vi "Vision on GIC Lab.vi"(11 "GIC Input":T2={"Real/Sim"=FALSE, "WP Lats and Longs"={"WP Lats"=[], "WP Longs"=[]}, "GPS Time Int"=0.0, "GPS Com Port"="", "Compass Com Port"="", "Prop Com Port"="", "GPS Data"=[], "Compass"=0.0, "LMS Vector"=[], "Vision Vector"=[], "Direction Cmd"=0.0, "Speed Cmd"=0.0, "Time of Last GPS"=0.0, "WP Vector"=[], "WP Number"=0, "Num of WPs"=0, "SW Map"=[], "Obst Lats and Longs"={"Obst Lats"=[], "Obst Longs"=[]}, "Parameters"=[], "Path Cluster"={"Path x nodes"=[], "Path y nodes"=[]}, "     Use ?\nOff       On"=[TRUE, TRUE, FALSE, FALSE]} {"Obst Lats and Longs"."Obst Longs" format="%#_8g"; "Obst Lats and Longs"."Obst Lats" format="%#_8g"}) -> (3 "GIC Output":T2={"Real/Sim"=FALSE, "WP Lats and Longs"={"WP Lats"=[], "WP Longs"=[]}, "GPS Time Int"=0.0, "GPS Com Port"="", "Compass Com Port"="", "Prop Com Port"="", "GPS Data"=[], "Compass"=0.0, "LMS Vector"=[], "Vision Vector"=[], "Direction Cmd"=0.0, "Speed Cmd"=0.0, "Time of Last GPS"=0.0, "WP Vector"=[], "WP Number"=0, "Num of WPs"=0, "SW Map"=[], "Obst Lats and Longs"={"Obst Lats"=[], "Obst Longs"=[]}, "Parameters"=[], "Path Cluster"={"Path x nodes"=[], "Path y nodes"=[]}, "     Use ?\nOff       On"=[TRUE, TRUE, FALSE, FALSE]} {"Obst Lats and Longs"."Obst Longs" format="%#_8g"; "Obst Lats and Longs"."Obst Lats" format="%#_8g"})   [LabVIEW 2014]
panel:
  out "Image Out":T1(plugin-control)
  out "swmap":dbl[][](array[numeric])
  # "Vision on GIC"
  # "GPS"
  # "LMS"
  # "Vision"
  # "Prop"
  # "GPS"
  # "LMS"
  # "Vision"
  # "Prop"
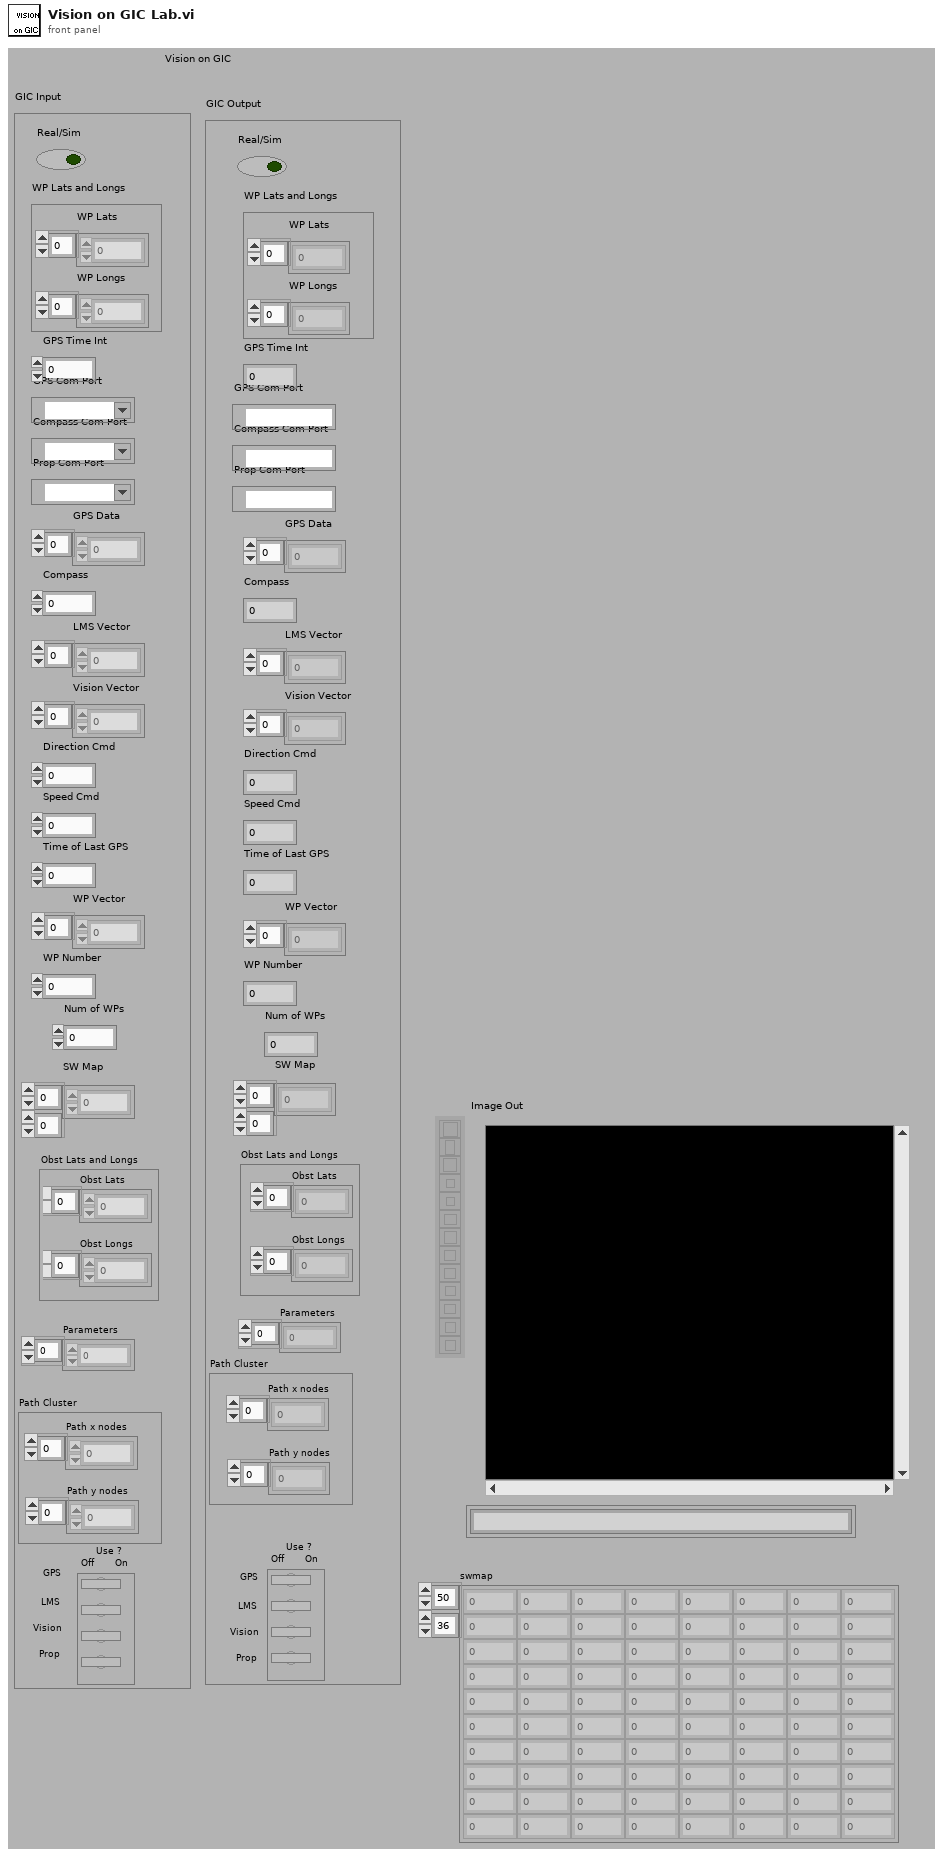
[diagram p1: front panel]
types:
  T1 = typedef "IMAQ Image.ctl" = refnum<image>
  T2 = cluster{"Real/Sim":bool, "WP Lats and Longs":cluster{"WP Lats":dbl[], "WP Longs":dbl[]}, "GPS Time Int":dbl, "GPS Com Port":refnum<visa-resource-name>, "Compass Com Port":refnum<visa-resource-name>, "Prop Com Port":refnum<visa-resource-name>, "GPS Data":dbl[], "Compass":dbl, "LMS Vector":dbl[], "Vision Vector":dbl[], "Direction Cmd":dbl, "Speed Cmd":dbl, "Time of Last GPS":dbl, "WP Vector":dbl[], "WP Number":i32, "Num of WPs":i16, "SW Map":i32[][], "Obst Lats and Longs":cluster{"Obst Lats":dbl[], "Obst Longs":dbl[]}, "Parameters":dbl[], "Path Cluster":cluster{"Path x nodes":dbl[], "Path y nodes":dbl[]}, "     Use ?\nOff       On":bool[]}
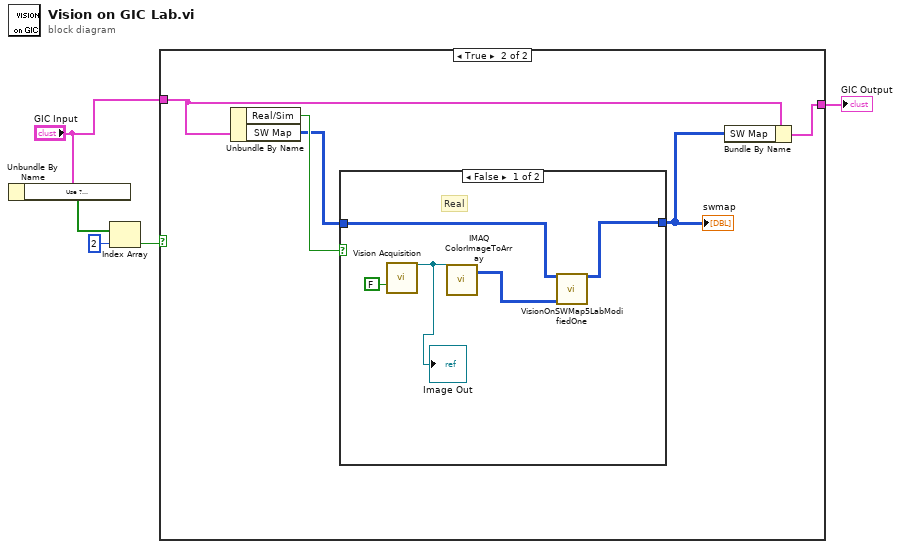
[diagram p0: block diagram]
diagram:
  n1 = Unbundle By Name("GIC Input") -> ("Use ?\nOff       On"=w5:bool[])
  n2 = Index Array(array=w5, index=2) -> (element=w1:bool)
  n3 = case shown="True" w1 {
    tunnel: "GIC Input" -> [w6 w10]
    tunnel: [w6 w8] -> w2
    frame False {
    }
    frame True {
      n4 = Unbundle By Name(w10) -> ("Real/Sim"=w11:bool, "SW Map"=w7:i32[][])
      n5 = case shown="False" w11 {
        tunnel: w7 -> [w15 w17]
        tunnel: [w13 w17] -> w9
        frame False {
          # "Real"
          n6 = call "Vision Acquisition"("Stop (F)"=FALSE) -> ("Image Out"=w12:T1)  [unwired: 24 in, 2 out]
          "Image Out" <- w12
          n7 = call "IMAQ ColorImageToArray"("Image"=w12) -> ("Image Pixels (U32)"=w16:u32[][])  [unwired: 3 in, 2 out]
          n8 = call "VisionOnSWMap5LabModifiedOne.vi"("SWMap In"=w15, "Image Pixels"=w16) -> ("SWMap Out"=w13:i32[][])  [unwired: 13 in]
        }
        frame True {
          # "Sim"
        }
      }
      "swmap" <- w9
      n9 = Bundle By Name(cluster=w10, "SW Map"=w9) -> (w8:T2)
    }
  }
  "GIC Output" <- w2
